vi "7.4.-Realidad Virtual - Estereoscopio.vi"() -> ()   [LabVIEW 2020]
uses:
  <vilib>/userDefined/High Color/IMAQdx.ctl
  <vilib>/Utility/miscctls.llb/LV3DPointTypeDef.ctl
  7.1.-ENUM Estereoscopio.ctl
  <vilib>/vision/Image Controls.llb/IMAQ Image.ctl
  60b5eb36-2a53-4617-8dfa-5e3f653ce4d9.vi
  <vilib>/picture/3D Picture Control/Object/Create Object (drawable).vi
  <vilib>/Comparison/Less/Less Functor/Less Functor.lvclass
  <vilib>/vision/driver/NI_Vision_Acquisition_Software.lvlib
  <vilib>/picture/3D Picture Control/NI_3D Picture Control.lvlib
panel:
  in  "f = Foco":dbl=455.0 format="%#_13g"
  in  "d = Distancia de Separación entre Cámaras":dbl=6.35 format="%#_13g"
  in  "Detener entorno virtual":bool
  out "X azul":dbl
  out "X verde":dbl
  out "X rojo":dbl
  out "Z azul":dbl
  out "Z verde":dbl
  out "Z rojo":dbl
  out "3":string
  out "2":string
  out "1":string
  in  "CONO VERDE":u32(colorbox)=1703680
  out "3D Picture":refnum<vi>(3d-picture)
  in  "CILINDRO AZUL":u32(colorbox)=393471
  in  "CUBO ROJO":u32(colorbox)=16711680
  in  "Color Eje XYZ":u32(colorbox)=16775680
  in  "Virtual Environment Perspective":T1={"X"=30.0, "Y"=15.0, "Z"=-40.0}
  in  "Detener todo":bool
  out "Cámara":T2(plugin-control)
  in  "Session In":T3="cam2"
  in  "Captura izquierda":bool
  in  "Captura derecha":bool
  # "Visión Artificial - Realidad Virtual - Estereoscopio\nDiego Cervantes Rodríguez\ndicer0.com"
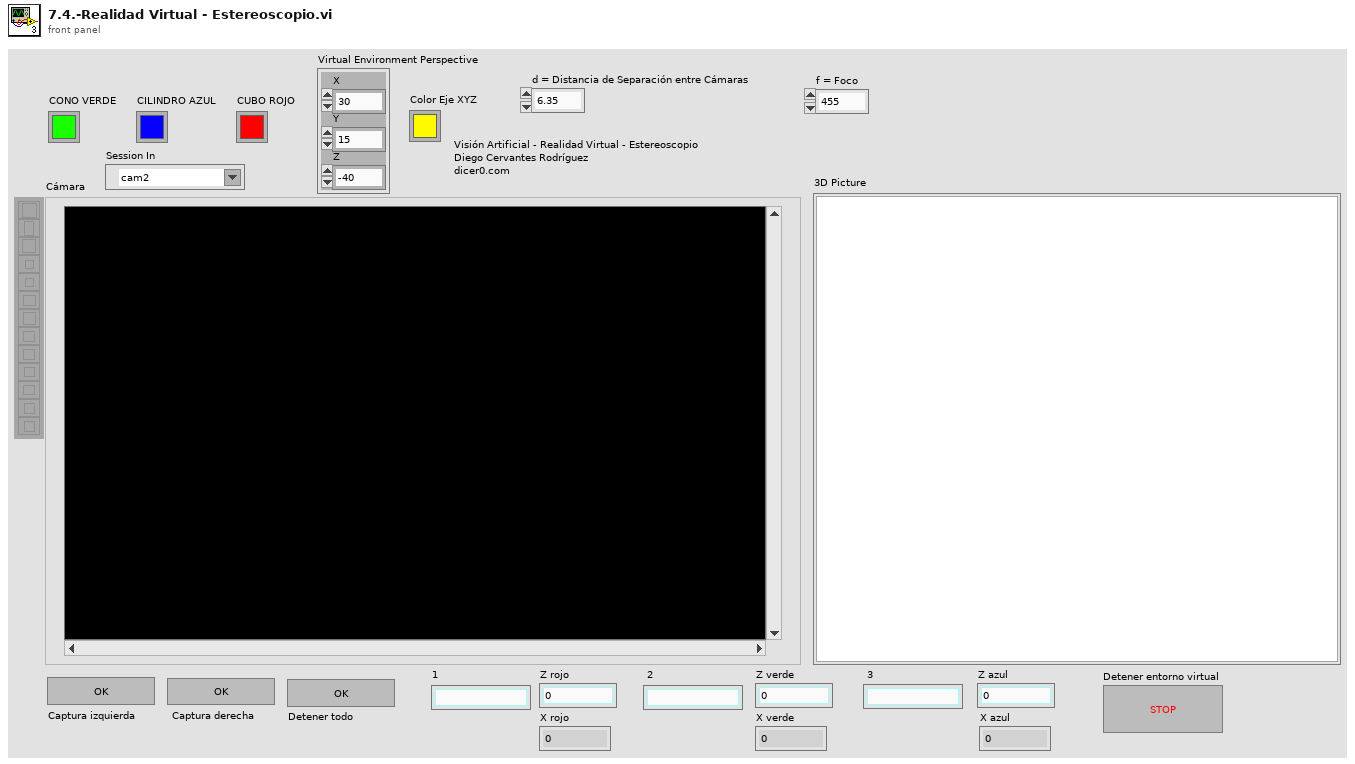
[diagram p1: front panel]
types:
  T1 = typedef "LV3DPointTypeDef.ctl" = cluster{"X":sgl, "Y":sgl, "Z":sgl}
  T2 = typedef "IMAQ Image.ctl" = refnum<image>
  T3 = typedef "IMAQdx.ctl" = refnum<k21>
  T4 = cluster{"DISTANCIAS":cluster{dbl, dbl, dbl, dbl, dbl, dbl}, "New Image":T2, "Session Out":T3, "IMAGENES":path[], "Image Out":T2, "error out":errorcluster}
  T5 = typedef "7.1.-ENUM Estereoscopio.ctl" = enum16{"Inicializar camara", "Mostrar plano virtual ", "Calculo de distancias", "Tomar foto der", "Tomar foto izq", "Espera"}
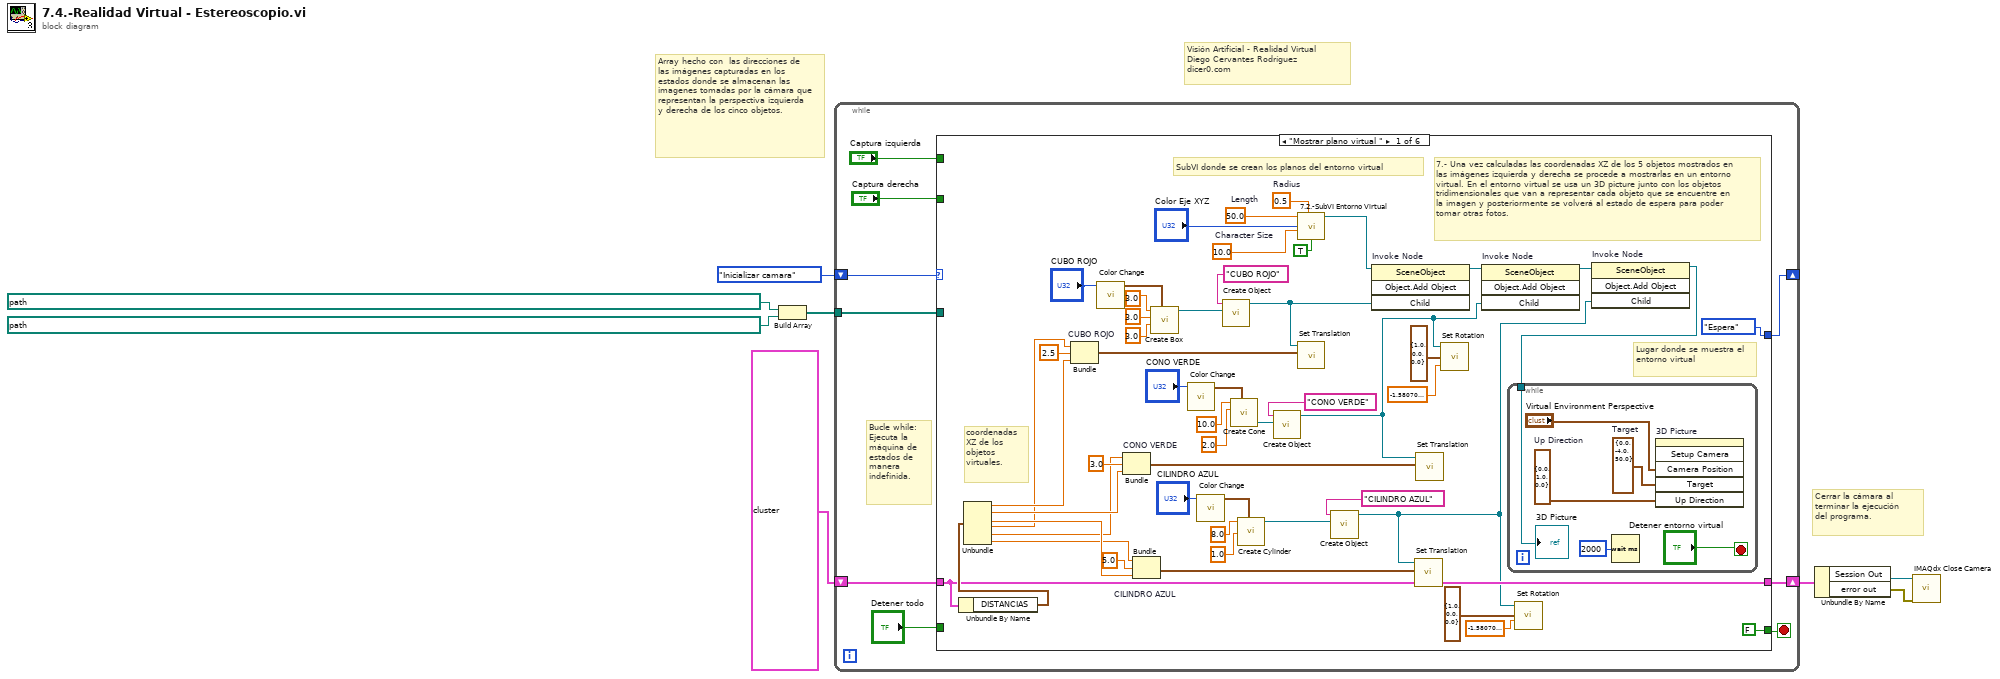
[diagram p0: block diagram]
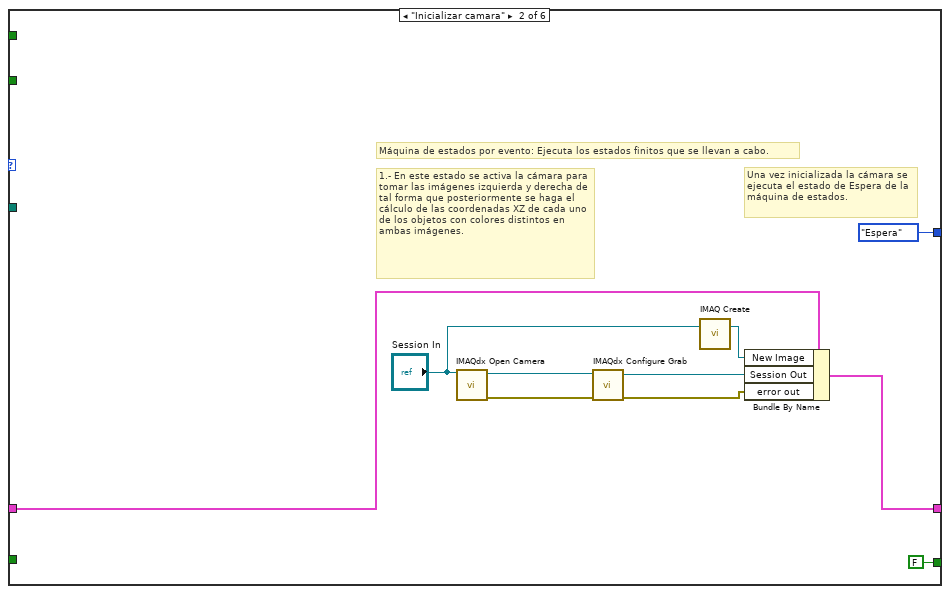
[diagram p2: hidden frame]
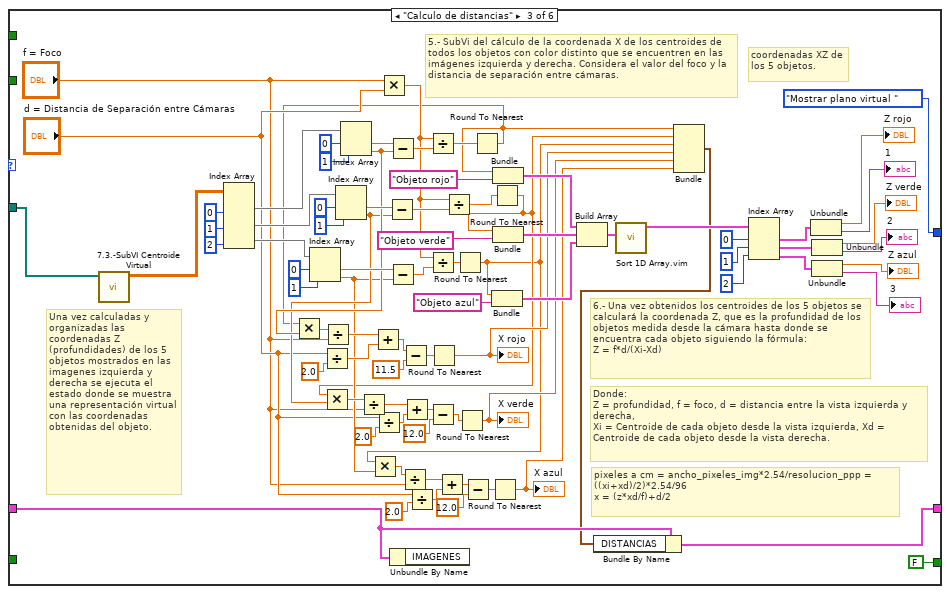
[diagram p3: hidden frame]
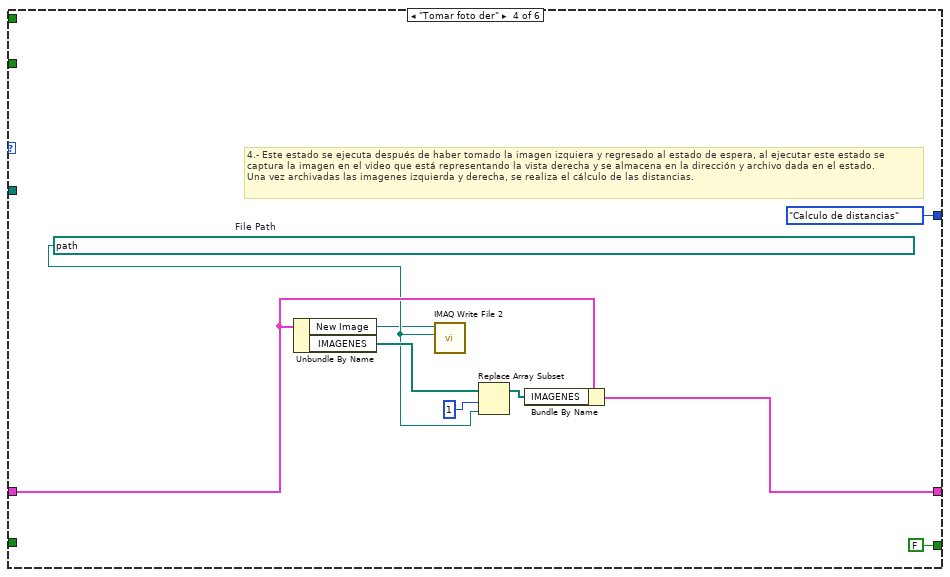
[diagram p4: hidden frame]
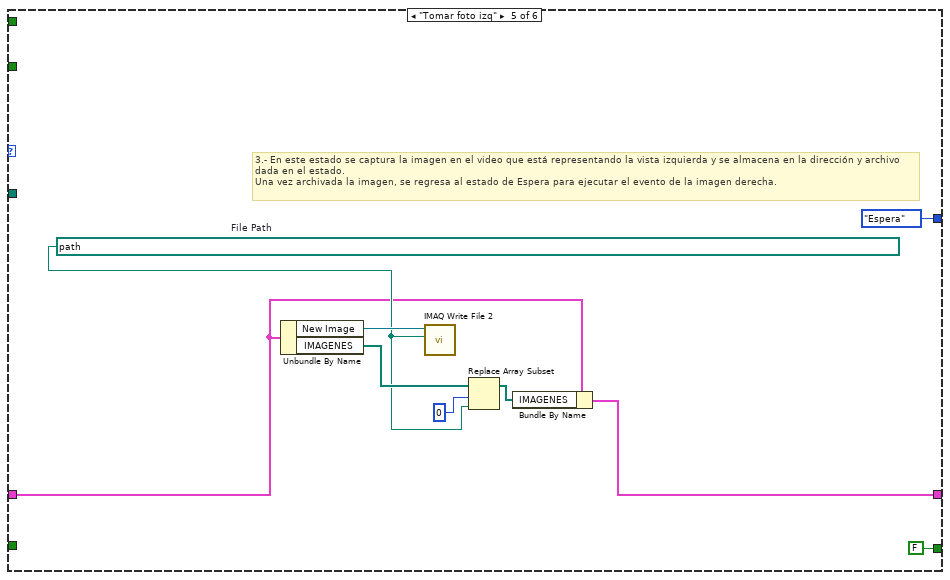
[diagram p5: hidden frame]
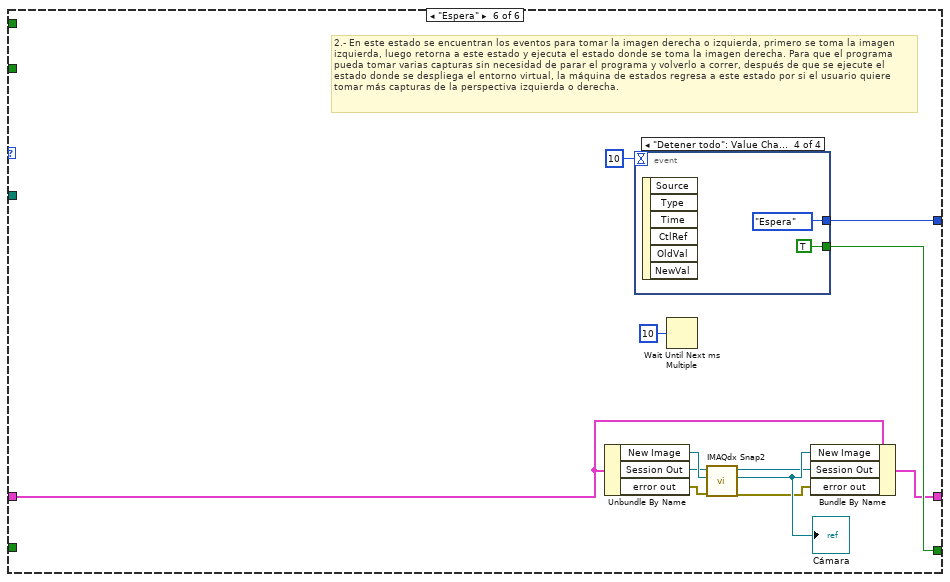
[diagram p6: hidden frame]
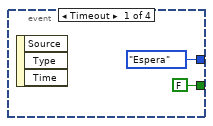
[diagram p7: hidden frame]
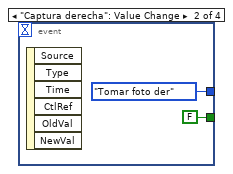
[diagram p8: hidden frame]
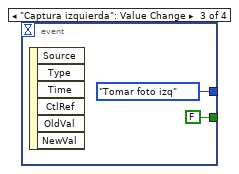
[diagram p9: hidden frame]
diagram:
  # "Array hecho con  las direcciones de las imágenes capturadas en los estados donde se almacenan las imagenes tomadas por la cámara que representan la perspectiva izquierda y derecha de los cinco objetos."
  # "Cerrar la cámara al terminar la ejecución del programa."
  # "Visión Artificial - Realidad Virtual\nDiego Cervantes Rodríguez\ndicer0.com"
  n1 = Build Array "Build Array"(path "C:/Users/diego/OneDrive/Documents/The_MechaBible/p_LabVIEW_ESP/1.-Sistemas de Visión Artificial/Img/7.0.-Realidad Virtual - Estereoscopio/fotoizq.png" ("File Path"), path "C:/Users/diego/OneDrive/Documents/The_MechaBible/p_LabVIEW_ESP/1.-Sistemas de Visión Artificial/Img/7.0.-Realidad Virtual - Estereoscopio/fotoder.png" ("File Path")) -> (w5:path[])
  n2 = while {
    shift-right: [w16] -> _
    shift-left: 7.1.-ENUM_Estereoscopio."Inicializar camara" -> [w17]
    tunnel: w5 -> [w12]
    shift-right: [w9] -> w3
    shift-left: T4 {"DISTANCIAS"={0.0, 0.0, 0.0, 0.0, 0.0, 0.0}, "New Image"=refnum, "Session Out"="", "IMAGENES"=[path "0", path "0"], "Image Out"=refnum, "error out"={"status"=FALSE, "code"=0, "source"=""}} -> [w10]
    stop <- w15 stop-if-true
    # "Bucle while: Ejecuta la máquina de estados de manera indefinida."
    n3 = case shown="\"Mostrar plano virtual \"" w17 {
      tunnel: [7.1.-ENUM_Estereoscopio."Espera" 7.1.-ENUM_Estereoscopio."Espera" 7.1.-ENUM_Estereoscopio."Mostrar plano virtual " 7.1.-ENUM_Estereoscopio."Calculo de distancias" 7.1.-ENUM_Estereoscopio."Espera" w195] -> w16
      tunnel: [FALSE FALSE FALSE FALSE FALSE w194] -> w15
      tunnel: "Captura izquierda" -> [_ _ _ _ _ _]
      tunnel: "Captura derecha" -> [_ _ _ _ _ _]
      tunnel: w12 -> [_ _ w130 _ _ _]
      tunnel: "Detener todo" -> [_ _ _ _ _ _]
      tunnel: w10 -> [w67 w79 w134 w172 w177 w184]
      tunnel: [w67 w75 w132 w167 w175 w186] -> w9
      frame "Mostrar plano virtual " {
        w61 = sgl 0.5  # Radius
        w60 = sgl 50.0  # Length
        w63 = sgl 10.0  # Character Size
        # "SubVI donde se crean los planos del entorno virtual"
        # "coordenadas XZ de los objetos virtuales."
        # "7.- Una vez calculadas las coordenadas XZ de los 5 objetos mostrados en las imágenes izquierda y derecha se procede a mostrarlas en un entorno virtual. En el entorno virtual se usa un 3D picture junto con los objetos tridimensionales que van a representar cada objeto que se encuentre en la imagen y posteriormente se volverá al estado de espera para poder tomar otras fotos."
        # "Lugar donde se muestra el entorno virtual"
        n4 = Unbundle By Name(w67) -> ("DISTANCIAS"=w68:cluster{dbl, dbl, dbl, dbl, dbl, dbl})
        n5 = Unbundle "Unbundle"(w68) -> (w24:dbl, w23:dbl, w22:dbl, w21:dbl, w20:dbl, w19:dbl)
        n6 = Bundle "CUBO ROJO"(w21, 2.5, w24) -> (w51:cluster{dbl, dbl, dbl})  [unwired: 1 in]
        n7 = call <vilib>:"Color Change.vi"("Color"="CUBO ROJO") -> ("RGBA"=w57:cluster{"R":sgl, "G":sgl, "B":sgl, "A":sgl})  [unwired: 10 in]
        n8 = Bundle "CONO VERDE"(w20, 3.0, w23) -> (w33:cluster{dbl, dbl, dbl})  [unwired: 1 in]
        n9 = Bundle "CILINDRO AZUL"(w19, 5.0, w22) -> (w40:cluster{dbl, dbl, dbl})  [unwired: 1 in]
        n10 = call <vilib>:"Create Box.vi"("Color"=w57, "Length Z"=sgl 3.0, "Length Y"=sgl 3.0, "Length X"=sgl 3.0) -> ("New Box Refnum"=w58:refnum<vi>)  [unwired: 6 in, 1 out]
        n11 = call <vilib>:"Color Change.vi"("Color"="CONO VERDE") -> ("RGBA"=w37:cluster{"R":sgl, "G":sgl, "B":sgl, "A":sgl})  [unwired: 10 in]
        n12 = call <vilib>:"Color Change.vi"("Color"="CILINDRO AZUL") -> ("RGBA"=w45:cluster{"R":sgl, "G":sgl, "B":sgl, "A":sgl})  [unwired: 10 in]
        n13 = call-poly <vilib>:"Create Object.vi"("Geometry"=w58, "Name"="CUBO ROJO") -> ("Scene:New Object"=w52:refnum<vi>)  [unwired: 8 in, 1 out]
        n14 = call <vilib>:"Create Cone.vi"("Color"=w37, "Radius"=sgl 2.0, "Height"=sgl 10.0) -> ("New Cone Refnum"=w39:refnum<vi>)  [unwired: 7 in, 1 out]
        n15 = call <vilib>:"Create Cylinder.vi"("Color"=w45, "Radius"=sgl 1.0, "Height"=sgl 8.0) -> ("New Cylinder Refnum"=w47:refnum<vi>)  [unwired: 7 in, 1 out]
        n16 = call-poly <vilib>:"Create Object.vi"("Geometry"=w39, "Name"="CONO VERDE") -> ("Scene:New Object"=w29:refnum<vi>)  [unwired: 8 in, 1 out]
        n17 = call "7.2.-SubVI Entorno Virtual.vi"("Axis label?"=TRUE, "Radius"=w61, "Character Size"=w63, "COLOR EJE XYZ"="Color Eje XYZ", "Length"=w60) -> ("SceneObject out"=w18:refnum<vi>)  [unwired: 6 in]
        n18 = call <vilib>:"Set Translation.vi"("Translation"=w51, "Scene Object"=w52) -> ()  [unwired: 8 in, 2 out]
        n19 = call-poly <vilib>:"Create Object.vi"("Geometry"=w47, "Name"="CILINDRO AZUL") -> ("Scene:New Object"=w26:refnum<vi>)  [unwired: 8 in, 1 out]
        n20 = invoke on="Invoke Node" class="SceneObject" method="Object.Add Object"(reference=w18, "Child"=w52) -> (reference out=w49:refnum<vi>)  [unwired: 2 in, 3 out]
        n21 = call <vilib>:"Set Translation.vi"("Translation"=w40, "Scene Object"=w26) -> ()  [unwired: 8 in, 2 out]
        n22 = call <vilib>:"Set Translation.vi"("Translation"=w33, "Scene Object"=w29) -> ()  [unwired: 8 in, 2 out]
        n23 = call <vilib>:"Set Rotation.vi"("Angle"=sgl -1.5807, "Axis"=cluster{"X":sgl, "Y":sgl, "Z":sgl} {"X"=1.0, "Y"=0.0, "Z"=0.0}, "Scene Object"=w29) -> ()  [unwired: 7 in, 2 out]
        n24 = invoke on="Invoke Node" class="SceneObject" method="Object.Add Object"(reference=w49, "Child"=w29) -> (reference out=w48:refnum<vi>)  [unwired: 2 in, 3 out]
        n25 = call <vilib>:"Set Rotation.vi"("Angle"=sgl -1.5807, "Axis"=cluster{"X":sgl, "Y":sgl, "Z":sgl} {"X"=1.0, "Y"=0.0, "Z"=0.0}, "Scene Object"=w26) -> ()  [unwired: 7 in, 2 out]
        n26 = invoke on="Invoke Node" class="SceneObject" method="Object.Add Object"(reference=w48, "Child"=w26) -> (reference out=w25:refnum<vi>)  [unwired: 2 in, 3 out]
        n27 = while {
          tunnel: w25 -> [w70]
          stop <- "Detener entorno virtual" stop-if-true
          w71 = T1 {"X"=0.0, "Y"=1.0, "Z"=0.0}  # Up Direction
          w73 = T1 {"X"=0.0, "Y"=-4.0, "Z"=50.0}  # Target
          n28 = Wait (ms)(milliseconds to wait=u32 2000) -> ()  [unwired: 1 out]
          n29 = invoke on="3D Picture" class="SceneGraphDisp (strict)" method="Setup Camera"("Camera Position"="Virtual Environment Perspective", "Target"=w73, "Up Direction"=w71) -> ()  [unwired: 3 in, 6 out]
          "3D Picture" <- w70
        }
      }
      frame "Inicializar camara" {
        # "Una vez inicializada la cámara se ejecuta el estado de Espera de la máquina de estados."
        # "Máquina de estados por evento: Ejecuta los estados finitos que se llevan a cabo."
        # "1.- En este estado se activa la cámara para tomar las imágenes izquierda y derecha de tal forma que posteriormente se haga el cálculo de las coordenadas XZ de cada uno de los objetos con colores distintos en ambas imágenes."
        n30 = call <vilib>:"IMAQdx Open Camera.vi"("Session In"="Session In") -> ("error out"=w83:errorcluster, "Session Out"=w84:T3)  [unwired: 9 in]
        n31 = call <vilib>:"IMAQdx Configure Grab.vi"("error in"=w83, "Session In"=w84) -> ("error out"=w76:errorcluster, "Session Out"=w77:T3)  [unwired: 8 in]
        n32 = call "IMAQ Create"("Image Name"="Session In") -> ("New Image"=w78:T2)  [unwired: 4 in, 1 out]
        n33 = Bundle By Name "Bundle By Name"(cluster=w79, "New Image"=w78, "Session Out"=w77, "error out"=w76) -> (w75:T4)
      }
      frame "Calculo de distancias" {
        # "coordenadas XZ de los 5 objetos."
        # "Donde:\nZ = profundidad, f = foco, d = distancia entre la vista izquierda y derecha, \nXi = Centroide de cada objeto desde la vista izquierda, Xd = Centroide de cada objeto desde la vista derecha."
        # "6.- Una vez obtenidos los centroides de los 5 objetos se calculará la coordenada Z, que es la profundidad de los objetos medida desde la cámara hasta donde se encuentra cada objeto siguiendo la fórmula:\nZ = f*d/(Xi-Xd)"
        # "Una vez calculadas y organizadas las coordenadas Z (profundidades) de los 5 objetos mostrados en las imagenes izquierda y derecha se ejecuta el estado donde se muestra una representación virtual con las coordenadas obtenidas del objeto."
        # "5.- SubVi del cálculo de la coordenada X de los centroides de todos los objetos con color distinto que se encuentren en las imágenes izquierda y derecha. Considera el valor del foco y la distancia de separación entre cámaras."
        # "pixeles a cm = ancho_pixeles_img*2.54/resolucion_ppp =\n((xi+xd)/2)*2.54/96\nx = (z*xd/f)+d/2"
        n34 = call "7.3.-SubVI Centroide Virtual.vi"("Array 3"=w130) -> ("Array 2"=w135:dbl[][])  [unwired: 10 in]
        n35 = Index Array "Index Array"(array=w135, index (col) #1=0 ("disabled index (col)"), index (col) #2=1 ("index (col)"), index (col) #3=2 ("index (col)")) -> (element #1=w138:dbl[], element #2=w137:dbl[], element #3=w136:dbl[])  [unwired: 3 in]
        n36 = Index Array(array=w136, index #1=0 ("index"), index #2=1 ("index")) -> (element #1=w121:dbl, element #2=w106:dbl)
        n37 = Divide(x="d = Distancia de Separación entre Cámaras", y=2.0) -> (x/y=w117:dbl)
        n38 = Index Array(array=w137, index #1=0 ("index"), index #2=1 ("index")) -> (element #1=w122:dbl, element #2=w111:dbl)
        n39 = Index Array "Index Array"(array=w138, index #1=0 ("index"), index #2=1 ("index")) -> (element #1=w123:dbl, element #2=w120:dbl)
        n40 = Divide(x="d = Distancia de Separación entre Cámaras", y=2.0) -> (x/y=w116:dbl)
        n41 = Multiply(x="f = Foco", y="d = Distancia de Separación entre Cámaras") -> (x*y=w141:dbl)
        n42 = Subtract(x=w122, y=w111) -> (x-y=w157:dbl)
        n43 = Subtract(x=w123, y=w120) -> (x-y=w160:dbl)
        n44 = Subtract(x=w121, y=w106) -> (x-y=w140:dbl)
        n45 = Unbundle By Name "Unbundle By Name"(w134) -> ()  [unwired: 1 out]
        n46 = Divide(x="d = Distancia de Separación entre Cámaras", y=2.0) -> (x/y=w107:dbl)
        n47 = Divide(x=w141, y=w160) -> (x/y=w92:dbl)
        n48 = Divide(x=w141, y=w140) -> (x/y=w88:dbl)
        n49 = Divide(x=w141, y=w157) -> (x/y=w90:dbl)
        n50 = Round To Nearest(number=w88) -> (nearest integer value=w87:dbl)
        n51 = Multiply(x=w87, y=w106) -> (x*y=w110:dbl)
        n52 = Divide(x=w110, y="f = Foco") -> (x/y=w108:dbl)
        n53 = Add(x=w108, y=w107) -> (x+y=w99:dbl)
        n54 = Subtract(x=w99, y=12.0) -> (x-y=w97:dbl)
        n55 = Round To Nearest(number=w92) -> (nearest integer value=w91:dbl)
        n56 = Multiply(x=w91, y=w120) -> (x*y=w119:dbl)
        n57 = Divide(x=w119, y="f = Foco") -> (x/y=w118:dbl)
        n58 = Add(x=w118, y=w117) -> (x+y=w104:dbl)
        n59 = Subtract(x=w104, y=11.5) -> (x-y=w96:dbl)
        n60 = Round To Nearest(number=w96) -> (nearest integer value=w93:dbl)
        "X rojo" <- w93
        n61 = Round To Nearest(number=w97) -> (nearest integer value=w95:dbl)
        "X azul" <- w95
        n62 = Round To Nearest(number=w90) -> (nearest integer value=w89:dbl)
        n63 = Multiply(x=w89, y=w111) -> (x*y=w113:dbl)
        n64 = Divide(x=w113, y="f = Foco") -> (x/y=w115:dbl)
        n65 = Add(x=w115, y=w116) -> (x+y=w102:dbl)
        n66 = Subtract(x=w102, y=12.0) -> (x-y=w98:dbl)
        n67 = Round To Nearest(number=w98) -> (nearest integer value=w94:dbl)
        "X verde" <- w94
        n68 = Bundle "Bundle"(w87, "Objeto azul") -> (w149:cluster{dbl, string})  [unwired: 1 in]
        n69 = Bundle(w91, "Objeto rojo") -> (w147:cluster{dbl, string})  [unwired: 1 in]
        n70 = Bundle(w89, "Objeto verde") -> (w148:cluster{dbl, string})  [unwired: 1 in]
        n71 = Build Array "Build Array"(w147, w148, w149) -> (w154:cluster{dbl, string}[])
        n72 = call "Sort 1D Array.vim"("unsorted array"=w154) -> ("sorted array"=w153:cluster{dbl, string}[])  [unwired: 10 in]
        n73 = Bundle "Bundle"(w91, w89, w87, w93, w94, w95) -> (w133:cluster{dbl, dbl, dbl, dbl, dbl, dbl})  [unwired: 1 in]
        n74 = Bundle By Name "Bundle By Name"(cluster=w134, "DISTANCIAS"=w133) -> (w132:T4)
        n75 = Index Array "Index Array"(array=w153, index #1=0 ("index"), index #2=1 ("index"), index #3=2 ("index")) -> (element #1=w144:cluster{dbl, string}, element #2=w143:cluster{dbl, string}, element #3=w142:cluster{dbl, string})
        n76 = Unbundle(w144) -> (→"Z rojo":dbl, →"1":string)
        n77 = Unbundle(w143) -> (→"Z verde":dbl, →"2":string)
        n78 = Unbundle "Unbundle"(w142) -> (→"Z azul":dbl, →"3":string)
      }
      frame "Tomar foto der" {
        w169 = path "C:/Users/diego/OneDrive/Documents/The_MechaBible/p_LabVIEW_ESP/1.-Sistemas de Visión Artificial/Img/7.0.-Realidad Virtual - Estereoscopio/fotoder.png"  # File Path
        # "4.- Este estado se ejecuta después de haber tomado la imagen izquiera y regresado al estado de espera, al ejecutar este estado se captura la imagen en el video que está representando la vista derecha y se almacena en la dirección y archivo dada en el estado.\nUna vez archivadas las imagenes izquierda y derecha, se realiza el cálculo de las distancias."
        n79 = Unbundle By Name "Unbundle By Name"(w172) -> ("New Image"=w166:T2, "IMAGENES"=w171:path[])
        n80 = call-poly "IMAQ Write File 2"("File Path"=w169, "Image"=w166) -> ()  [unwired: 8 in, 2 out]
        n81 = Replace Array Subset "Replace Array Subset"(array=w171, new element=w169, index=1) -> (w168:path[])
        n82 = Bundle By Name "Bundle By Name"(cluster=w172, "IMAGENES"=w168) -> (w167:T4)
      }
      frame "Tomar foto izq" {
        w178 = path "C:/Users/diego/OneDrive/Documents/The_MechaBible/p_LabVIEW_ESP/1.-Sistemas de Visión Artificial/Img/7.0.-Realidad Virtual - Estereoscopio/fotoizq.png"  # File Path
        # "3.- En este estado se captura la imagen en el video que está representando la vista izquierda y se almacena en la dirección y archivo dada en el estado.\nUna vez archivada la imagen, se regresa al estado de Espera para ejecutar el evento de la imagen derecha."
        n83 = Unbundle By Name "Unbundle By Name"(w177) -> ("New Image"=w181:T2, "IMAGENES"=w180:path[])
        n84 = call-poly "IMAQ Write File 2"("File Path"=w178, "Image"=w181) -> ()  [unwired: 8 in, 2 out]
        n85 = Replace Array Subset "Replace Array Subset"(array=w180, new element=w178, index=0) -> (w176:path[])
        n86 = Bundle By Name "Bundle By Name"(cluster=w177, "IMAGENES"=w176) -> (w175:T4)
      }
      frame "Espera" {
        # "2.- En este estado se encuentran los eventos para tomar la imagen derecha o izquierda, primero se toma la imagen izquierda, luego retorna a este estado y ejecuta el estado donde se toma la imagen derecha. Para que el programa pueda tomar varias capturas sin necesidad de parar el programa y volverlo a correr, después de que se ejecute el estado donde se despliega el entorno virtual, la máquina de estados regresa a este estado por si el usuario quiere tomar más capturas de la perspectiva izquierda o derecha."
        n87 = Unbundle By Name "Unbundle By Name"(w184) -> ("New Image"=w192:T2, "Session Out"=w191:T3, "error out"=w190:errorcluster)
        n88 = event shown="[3] \"Detener todo\": Value Change" {
          selector: _ -> [_ _ _ _]
          dyn-events: _ -> [_ _ _ _]
          timeout: 10 -> [_ _ _ _]
          tunnel: [7.1.-ENUM_Estereoscopio."Espera" 7.1.-ENUM_Estereoscopio."Tomar foto der" 7.1.-ENUM_Estereoscopio."Tomar foto izq" 7.1.-ENUM_Estereoscopio."Espera"] -> w195
          tunnel: [FALSE FALSE FALSE TRUE] -> w194
          event Timeout {
            n89 = event-data() -> ()  [unwired: 1 in, 3 out]
          }
          event "Captura derecha": Value Change {
            n90 = event-data() -> ()  [unwired: 1 in, 6 out]
          }
          event "Captura izquierda": Value Change {
            n91 = event-data() -> ()  [unwired: 1 in, 6 out]
          }
          event "Detener todo": Value Change {
            n92 = event-data() -> ()  [unwired: 1 in, 6 out]
          }
        }
        n93 = Wait Until Next ms Multiple(millisecond multiple=u32 10) -> ()  [unwired: 1 out]
        n94 = call <vilib>:"IMAQdx Snap2.vi"("error in"=w190, "Image In"=w192, "Session In"=w191) -> ("error out"=w187:errorcluster, "Image Out"=w189:T2, "Session Out"=w188:T3)  [unwired: 6 in]
        "Cámara" <- w189
        n95 = Bundle By Name "Bundle By Name"(cluster=w184, "New Image"=w189, "Session Out"=w188, "error out"=w187) -> (w186:T4)
      }
    }
  }
  n96 = Unbundle By Name "Unbundle By Name"(w3) -> ("Session Out"=w2:T3, "error out"=w1:errorcluster)
  n97 = call <vilib>:"IMAQdx Close Camera.vi"("error in"=w1, "Session In"=w2) -> ()  [unwired: 9 in, 1 out]
